vi "Func_GetLvlibPath.vi"(8 "error in (no error)":errorcluster, 11 "VI in":refnum<vi>) -> (0 "error out":errorcluster, 3 "VI Path":path)   [LabVIEW 2010, in "TemplateGenerator.lvlib"]
uses:
  TemplateGenerator.lvlib
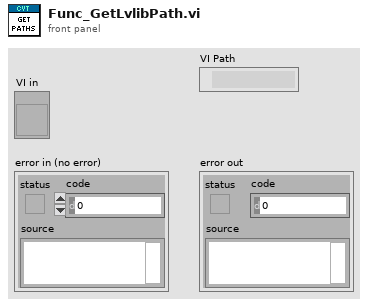
[diagram p1: front panel]
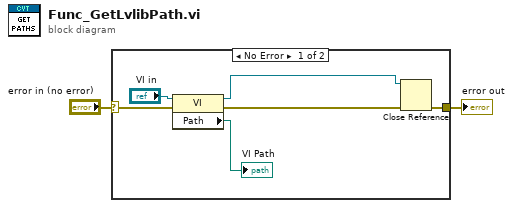
[diagram p0: block diagram]
diagram:
  n1 = case shown="No Error" "error in (no error)" {
    selector: "error in (no error)" -> [w5 w9]
    tunnel: [w7 w9] -> w2
    frame No Error {
      n2 = property class="VI"(reference="VI in", error in=w5) -> (reference out=w6:refnum<vi>, error out=w3:errorcluster, "Path"=→"VI Path":path)
      n3 = Close Reference(reference=w6, error in (no error)=w3) -> (error out=w7:errorcluster)
    }
    frame Error {
    }
  }
  "error out" <- w2
